vi "test_MultipleSessionsReserved_CallCreateSessions_SessionsAddedToConnectionMap.vi"(8 "error in":errorcluster) -> (0 "error out":errorcluster, 2 "result":string, 3 "pass":bool)   [LabVIEW 2020, in "MeasurementServerTests.lvlib"]
uses:
  MeasurementServerTests.lvlib
  Helpers/Fake Instrument/Fake Instrument.lvclass
  da6ffb6f-c1c9-4957-84dd-e9228483c454.vi
  a956f7ee-c7e9-4639-884c-f4265dae6ecf.vi
  Runtime/MeasurementLink Session Management/Session Reservation/Connection.ctl
  Runtime/MeasurementLink Session Management/Session Reservation/Session Reservation.lvclass
  Runtime/MeasurementLink Session Management/Session Reservation/Connection with Session.ctl
  9551059f-18af-4e23-b734-10739766adb6.vi
  Runtime/MeasurementLink Session Management/Session Reservation/Pin Type.ctl
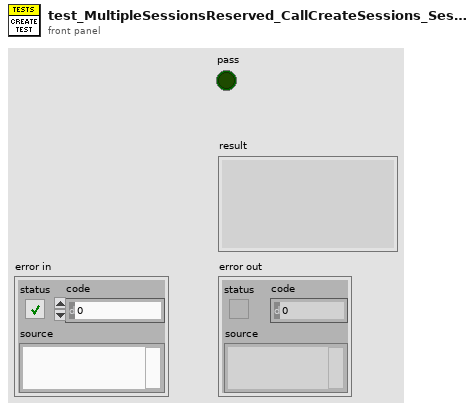
[diagram p1: front panel]
types:
  T1 = typedef "MeasurementLink Session Management.lvlib/Session Reservation.lvclass/Pin Type.ctl" = enum16{"All Pins", "DUT Pins", "System Pins"}
  T2 = typedef "MeasurementLink Session Management.lvlib/Session Reservation.lvclass/Connection with Session.ctl" = cluster{"connection":T3, "session":variant}
  T3 = typedef "MeasurementLink Session Management.lvlib/Session Reservation.lvclass/Connection.ctl" = cluster{"pin or relay name":string, "site":i32, "instrument type id":string, "channel":string}
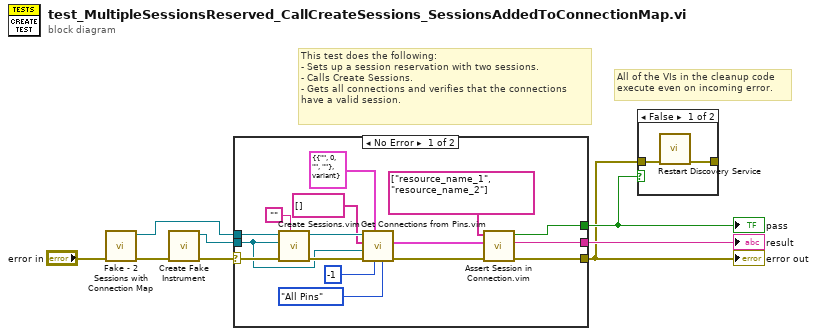
[diagram p0: block diagram]
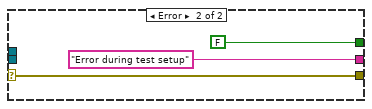
[diagram p2: hidden frame]
diagram:
  # "All of the VIs in the cleanup code\nexecute even on incoming error."
  # "This test does the following:\n- Sets up a session reservation with two sessions.\n- Calls Create Sessions.\n- Gets all connections and verifies that the connections\nhave a valid session."
  n1 = call "Fake - 2 Sessions with Connection Map.vi"("error in"="error in") -> ("error out"=w2:errorcluster, "session reservation out"=w1:refnum<class "Session Reservation.lvclass">)  [unwired: 9 in]
  n2 = call "Create Fake Instrument.vi"("error in"=w2) -> ("error out"=w5:errorcluster, "fake instrument out"=w4:refnum<class "Fake Instrument.lvclass">)  [unwired: 9 in]
  n3 = case shown="No Error" w5 {
    selector: w5 -> [w22 w24]
    tunnel: [w12 w24] -> w6
    tunnel: [w14 FALSE] -> w7
    tunnel: [w13 "Error during test setup" ("f")] -> w8
    tunnel: w4 -> [w17 _]
    tunnel: w1 -> [w23 _]
    frame No Error {
      n4 = call "Create Sessions.vim"("session type"="", "error in"=w22, "instrument"=w17, "session reservation in"=w23) -> ("error out"=w20:errorcluster, "session reservation out"=w19:refnum<class "Session Reservation.lvclass">)  [unwired: 4 in, 2 out]
      n5 = call "Get Connections from Pins.vim"("pin type"=Pin_Type."All Pins", "site"=-1, "connection type"=T2 {"connection"={"pin or relay name"="", "site"=0, "instrument type id"="", "channel"=""}, "session"=variant}, "error in"=w20, "instrument"=w17, "pin or relay names"=string[] [], "session reservation in"=w19) -> ("error out"=w12:errorcluster, "connections"=w11:T2[])  [unwired: 2 in, 1 out]
      n6 = call "Assert Session in Connection.vim"("actual connections"=w11, "expected session"=string[] ["resource_name_1", "resource_name_2"]) -> ("result"=w13:string, "pass"=w14:bool)  [unwired: 8 in]
    }
    frame Error {
    }
  }
  "error out" <- w6
  "pass" <- w7
  "result" <- w8
  n7 = case shown="False" w7 {
    tunnel: w6 -> [w28 _]
    tunnel: [w27 _] -> _
    frame False {
      n8 = call "Restart Discovery Service.vi"("error in"=w28) -> ("error out"=w27:errorcluster)  [unwired: 10 in]
    }
    frame True {
    }
  }
